vi "ReSample.vi"(9 "重采样率[Hz]":i32, 10 "原始采样率[Hz]":i32, 11 "原始数据":cluster{dbl[]}[](array[cluster])) -> (3 "重采样后数据":cluster{dbl[]}[](array[cluster]))   [LabVIEW 2018, in "DataDisplay.lvlib"]
uses:
  DataDisplay.lvlib
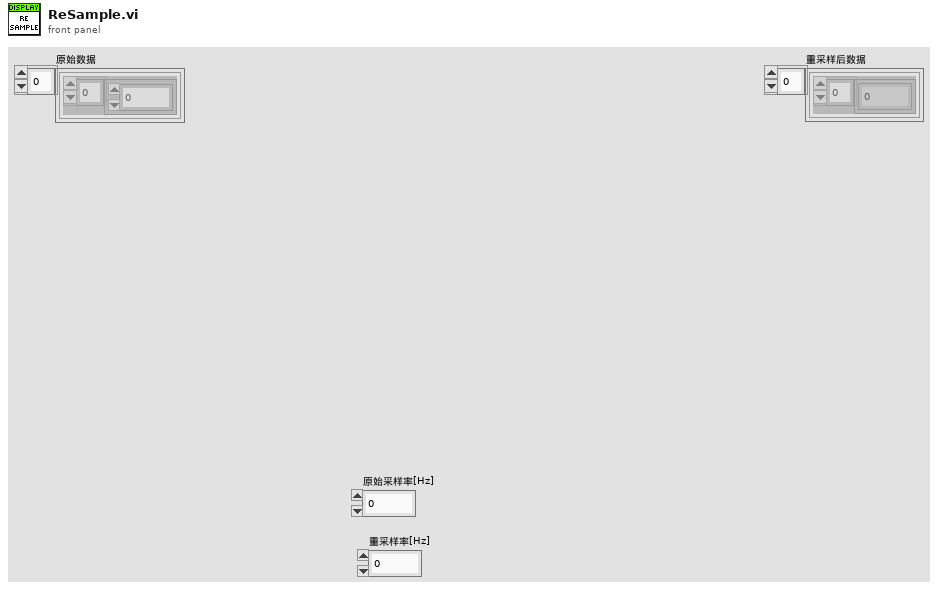
[diagram p1: front panel]
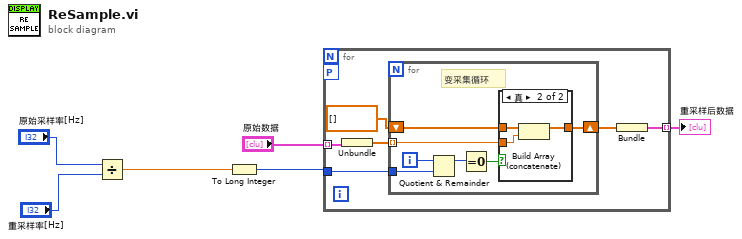
[diagram p0: block diagram]
diagram:
  n1 = Divide(x="原始采样率[Hz]", y="重采样率[Hz]") -> (x/y=w3:dbl)
  n2 = To Long Integer(number=w3) -> (32bit integer=w2:i32)
  n3 = for {
    tunnel: "原始数据" -> [w12] mode=indexing
    tunnel: [w10] -> w1 mode=indexing
    tunnel: w2 -> [w8]
    workers-P: _ -> [_]
    n4 = Unbundle(w12) -> (w7:dbl[])
    n5 = for {
      tunnel: w7 -> [w14] mode=indexing
      tunnel: w8 -> [w18]
      shift-right: [w13] -> w11
      shift-left: dbl[] [] -> [w15]
      i -> [w19]
      # "变采集循环"
      n6 = Quotient & Remainder(x=w19, y=w18) -> (x-y*floor(x/y)=w17:i32)  [unwired: 1 out]
      n7 = Equal To 0?(x=w17) -> (x = 0?=w16:bool)
      n8 = case shown="真" w16 {
        tunnel: w15 -> [w20 w23]
        tunnel: w14 -> [_ w22]
        tunnel: [w20 w21] -> w13
        frame False {
        }
        frame True {
          n9 = Build Array (concatenate)(w23, w22) -> (w21:dbl[])
        }
      }
    }
    n10 = Bundle(w11) -> (w10:cluster{dbl[]})  [unwired: 1 in]
  }
  "重采样后数据" <- w1
